vi "Init 5782.vi"(6 "Record length":u16, 7 "bitfile path":path, 8 "error in (no error)":errorcluster, 9 "Mode":T2, 10 "Device Name":refnum<k15>="RIO0", 11 "FPGA ref":T1) -> (0 "error out":errorcluster, 3 "FpgaRef5782 Out":refnum<class "FpgaRefx410.lvclass">)   [LabVIEW 2025, in "FpgaRefx410.lvclass"]
uses:
  FpgaRefx410.lvclass
  FPGA/DataMode.ctl
  x410 FPGA ref.ctl
  FPGA/fpga_settings.ctl
  FpgaRefx410.lvclass/FpgaRefx410.ctl
  <vilib>/Utility/error.llb/Error Cluster From Error Code.vi
  <vilib>/rvi/errors/niLvFpgaAdjustHostInterfaceError.vi
  <vilib>/rvi/interface/nirviReadWriteControl/nirviReadWriteControl.xnode
  FpgaRefBase/FpgaRefBase.lvclass
  NiFpgaLv.dll
  <vilib>/rvi/interface/Simulation/niFpgaSimulationCallBeginRW.vi
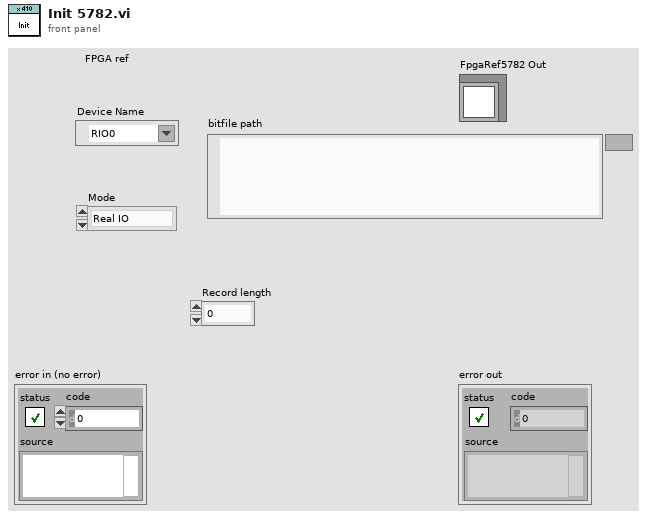
[diagram p1: front panel]
types:
  T1 = typedef "x410 FPGA ref.ctl" = refnum<k20>
  T2 = typedef "DataMode.ctl" = enum16{"Real IO", "Simulated"}
  T3 = typedef "fpga_settings.ctl" = enum16{"Feedback Enable", "New FIR coeffs", "FIR shift", "Enable filter", "Set Downsample", "Downsample", "CIC Gain", "Record length", "Trigger samples", "Quiet time", "a_am", "b_am", "Use fixed delay", "fixed sin_fi", "fixed cos_fi", "Ki*Tau", "Kp", "Kd_Tau", "Fi_start", "Fi_delta", "DC_offs 0", "DC_offs 1", "DC_offs 2", "DC_offs 3", "Ki*Tau am", "Kp am", "Kd_Tau am", "Feedback AM", "Trigger delay", "Feedback delay", "Setpoint enable", "Beam enable", "Samples to acquire", "Cavity Enable", "Cavity C1", "Cavity C2", "Cavity C3", "Cavity C4", "Cavity C5", "Input delay", "Ki*Tau Q", "Kp Q", "Kd_Tau Q", "Adaptive FF enable", "Feedforward a0", "Feedforward b0", "FF src adress", "FF dest adress", "Output scale", "Input scale", "Host scale", "FF_IIR b0", "FF_IIR b1", "FF_IIR b2", "FF_IIR-a1", "FF_IIR-a2", "Enable HW trigger", "Virtual cavity", "Samples to skip", "Samples to skip 2", "Samples to skip 3", "Cavity C3_2", "Cavity C4_2", "Cavity C5_2", "Cavity C3_3", "Cavity C4_3", "Cavity C5_3", "Cavity_w0_dt", "Piezo setting", "Quench t0", "Quench tau set", "Quench enabled", "Quench reset", "PID enabled I", "PID enabled Q", "Cavity filter a", "Cavity filter b", "Disable e(n)", "FF e(n) src address", "FF first address", "FF last address", "FF PID first address", "FF PID last address", "Amp IIR b0", "Amp IIR b1", "Amp IIR b2", "Amp IIR-a1", "Amp IIR-a2", "Adaptation factor", "Inv Amp LP b0", "Inv Amp LP b1", "Inv Amp LP b2", "Inv Amp LP-a1", "Inv Amp LP-a2", "Inv Amp c0", "Inv Amp c1", "Inv Amp c2", "Inv Amp c3", "Inv Amp c4", "Inv Amp -d1", "Inv Amp -d2", "Inv Amp -d3", "Inv Amp -d4", "w12_a", "w12_b", "w12_dt", "w12_scale", "dw_scale", "Extra output select", "Extra fi sin", "Extra fi cos", "Extra output scale", "Quench max output"}
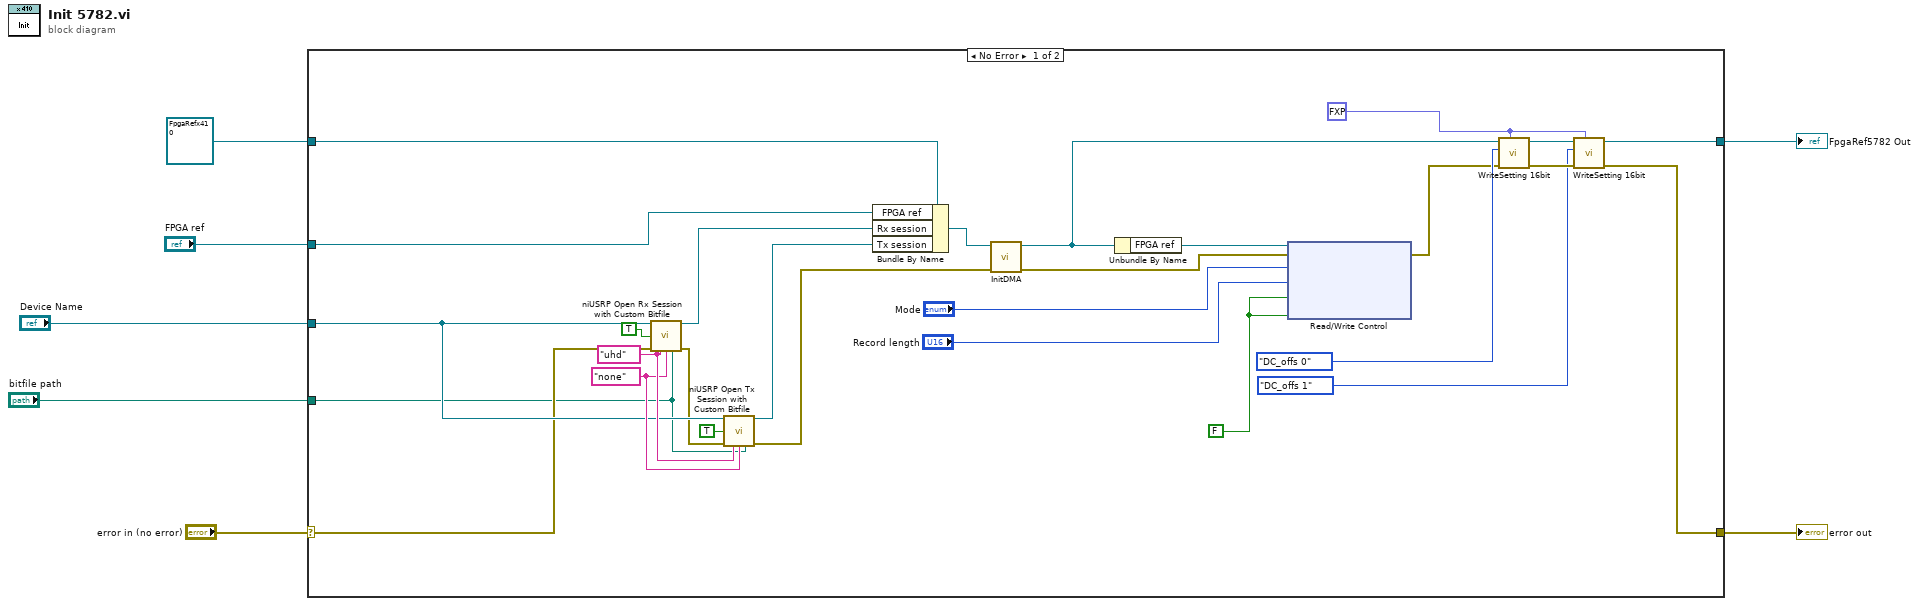
[diagram p0: block diagram]
diagram:
  n1 = case shown="No Error" "error in (no error)" {
    selector: "error in (no error)" -> [w14 w37]
    tunnel: [w20 w37] -> w6
    tunnel: [w24 w36] -> w5
    tunnel: refnum<class "FpgaRefx410.lvclass"> refnum ("FpgaRef5782 Out") -> [w34 w36]
    tunnel: "FPGA ref" -> [w10 _]
    tunnel: "bitfile path" -> [w11 _]
    tunnel: "Device Name" -> [w15 _]
    frame No Error {
      w17 = "none" ("streaming")
      w18 = "uhd" ("config")
      w26 = fxp<+,16,16> 0.0 ("value")
      w33 = FALSE
      n2 = call <instrlib>:"niUSRP Open Rx Session with Custom Bitfile.vi"("device names"=w15, "reset"=TRUE, "error in (no error)"=w14, "config"=w18, "streaming"=w17, "bitfile path"=w11) -> ("session handle out"=w9:refnum<k15>, "error out"=w13:errorcluster)  [unwired: 8 in]
      n3 = call <instrlib>:"niUSRP Open Tx Session with Custom Bitfile.vi"("device names"=w15, "reset"=TRUE, "error in (no error)"=w13, "config"=w18, "streaming"=w17, "bitfile path"=w11) -> ("session handle out"=w8:refnum<k15>, "error out"=w12:errorcluster)  [unwired: 8 in]
      n4 = Bundle By Name(cluster=w34, "FPGA ref"=w10, "Rx session"=w9, "Tx session"=w8) -> (w35:refnum<class "FpgaRefx410.lvclass">)
      n5 = call-dynamic "InitDMA.vi"("error in (no error)"=w12, "FpgaRef5782 in"=w35) -> ("error out"=w29:errorcluster, "FpgaRef5782 out"=w25:refnum<class "FpgaRefx410.lvclass">)  [unwired: 8 in]
      n6 = Unbundle By Name(w25) -> ("FPGA ref"=w32:T1)
      n7 = xnode "Read/Write Control"("FPGA VI Reference In"=w32, "error in"=w29, "Mode"="Mode", "Record length"="Record length", "Trigger Acquisition"=w33, "Acquisition running"=w33) -> ("error out"=w21:errorcluster)  [unwired: 1 out]
      n8 = call "WriteSetting 16bit.vi"("value"=w26, "error in (no error)"=w21, "FPGA Setting"=fpga_settings."DC_offs 0", "FpgaRefBase in"=w25) -> ("error out"=w27:errorcluster, "FpgaRefBase out"=w28:refnum<class "FpgaRefx410.lvclass">)  [unwired: 6 in]
      n9 = call "WriteSetting 16bit.vi"("value"=w26, "error in (no error)"=w27, "FPGA Setting"=fpga_settings."DC_offs 1", "FpgaRefBase in"=w28) -> ("error out"=w20:errorcluster, "FpgaRefBase out"=w24:refnum<class "FpgaRefx410.lvclass">)  [unwired: 6 in]
    }
    frame Error {
    }
  }
  "error out" <- w6
  "FpgaRef5782 Out" <- w5
